vi "Analyze_VIs.vi"(8 "error in (no error)":errorcluster) -> (0 "error out":errorcluster)   [LabVIEW 2020, in "AbCICD.lvlib"]
uses:
  AbCICD.lvlib
panel:
  in  "VI to analyze":path
  out "Summary Statistics":T1
  in  "ReportPath":path
  in  "VIANConfig":path
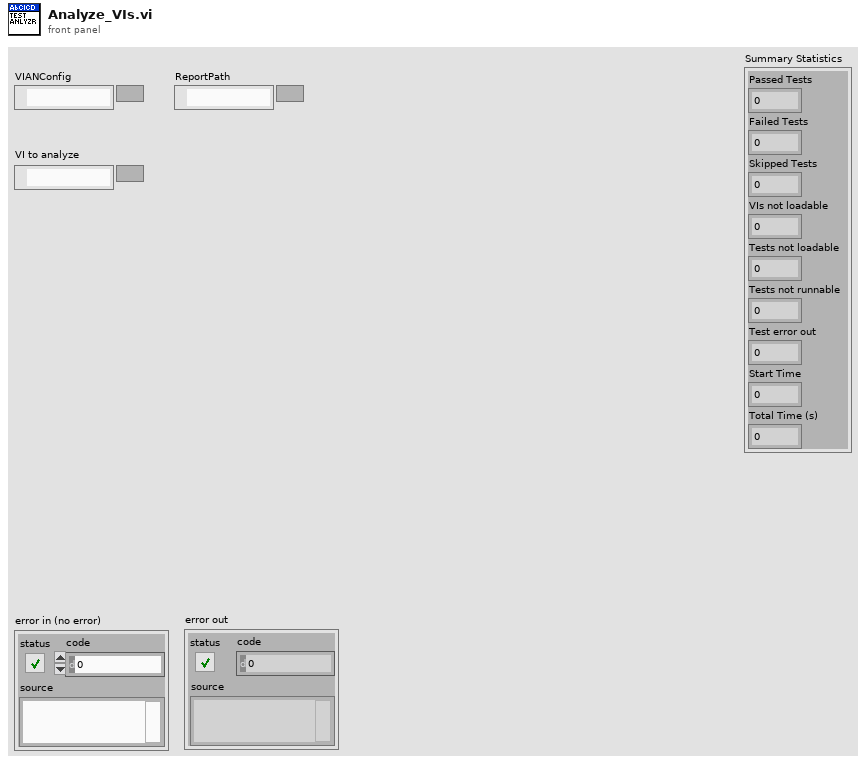
[diagram p1: front panel]
types:
  T1 = cluster{"Passed Tests":i32, "Failed Tests":i32, "Skipped Tests":i32, "VIs not loadable":i32, "Tests not loadable":i32, "Tests not runnable":i32, "Test error out":i32, "Start Time":u32, "Total Time (s)":dbl}
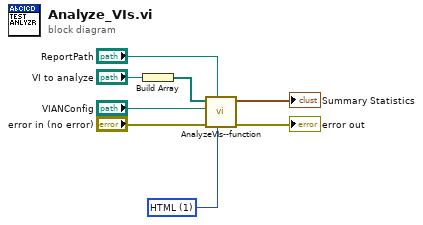
[diagram p0: block diagram]
diagram:
  w6 = u16 1 items=["ASCII", "HTML", "RSL File"] ("Report Save Type (ASCII)")
  n1 = Build Array("VI to analyze") -> (w1:path[])
  n2 = call "AnalyzeVIs--function.vi"("Report Save Type (ASCII)"=w6, "ReportPath"="ReportPath", "error in"="error in (no error)", "VIANConfig"="VIANConfig", "VIs to Analyze"=w1) -> ("error out"=→"error out":errorcluster, "Summary Statistics"=→"Summary Statistics":T1)  [unwired: 5 in]
